vi "RT.vi"() -> ()   [LabVIEW 2017]
panel:
  in  "Inject error":bool
  out "Numeric":i32
  out "Boolean":bool
  in  "stop":bool
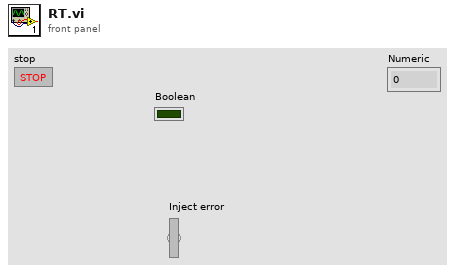
[diagram p1: front panel]
types:
  T1 = cluster{"source":string, "message":variant, "timestamp":timestamp}
  T2 = enum16{"open", "replace", "create", "open or create", "replace or create", "replace or create with confirmation"}
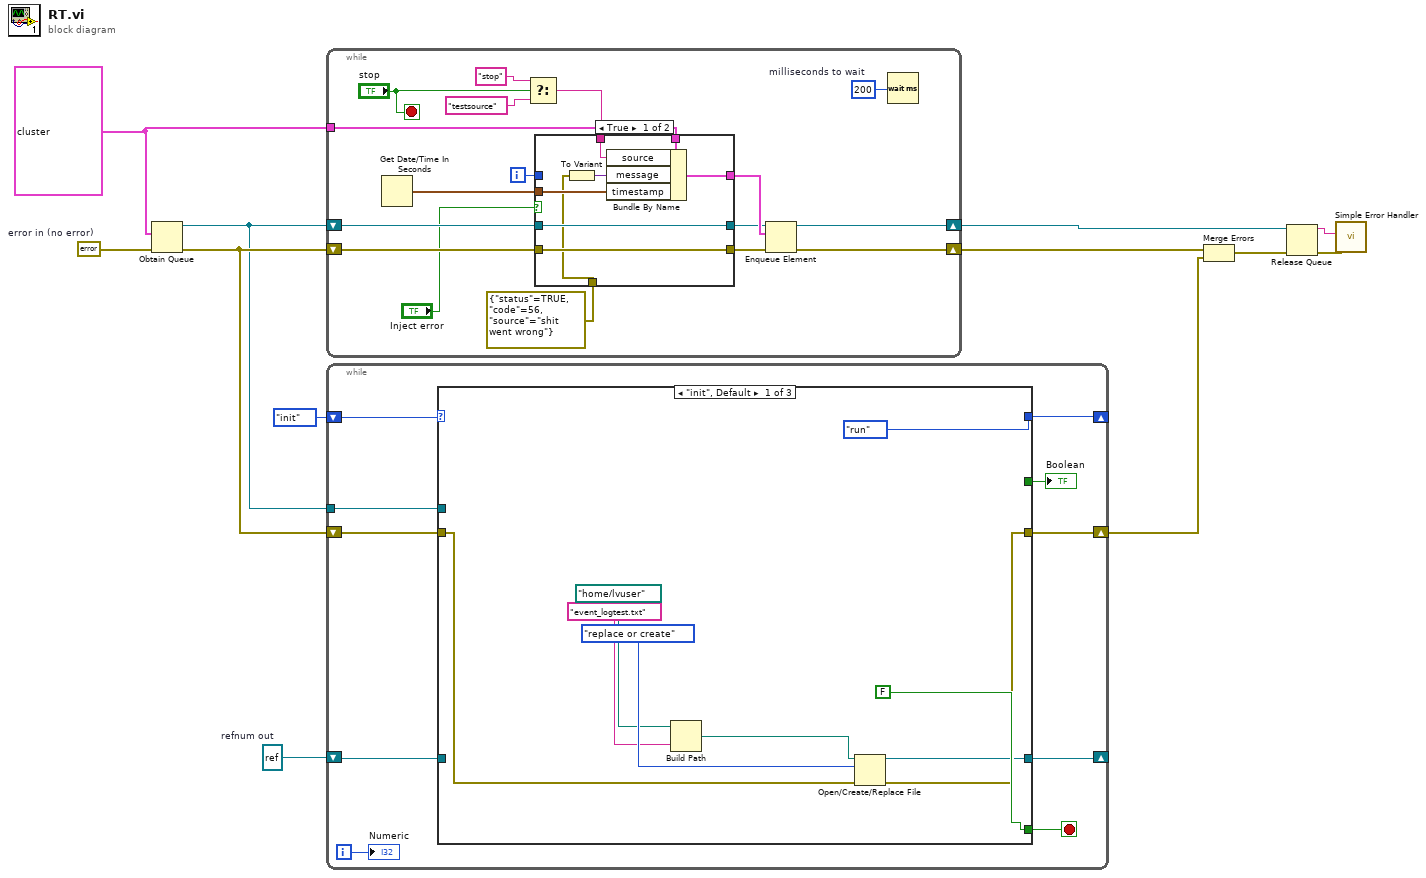
[diagram p0: block diagram]
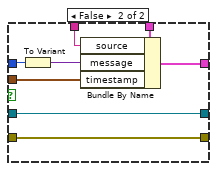
[diagram p2: hidden frame]
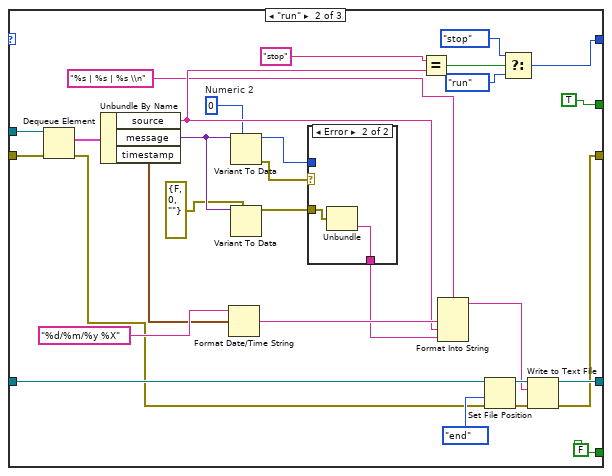
[diagram p3: hidden frame]
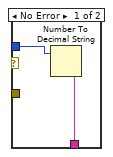
[diagram p4: hidden frame]
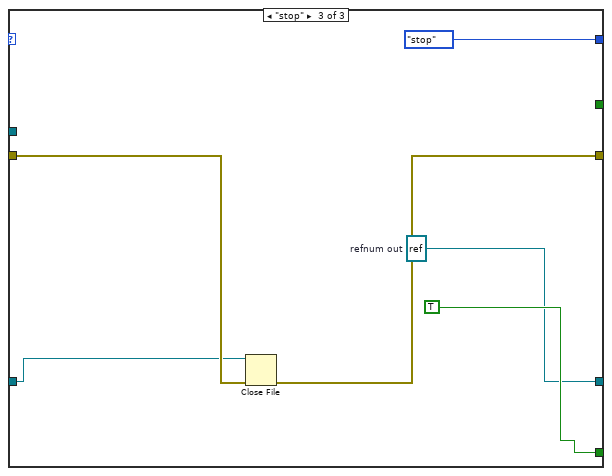
[diagram p5: hidden frame]
diagram:
  w7 = refnum<file> refnum  # refnum out
  w10 = T1 {"source"="", "message"=variant, "timestamp"=timestamp(0 s since 1904-01-01)}
  w12 = errorcluster {"status"=FALSE, "code"=0, "source"=""}  # error in (no error)
  n1 = Obtain Queue(element data type=w10, error in (no error)=w12) -> (queue out=w8:refnum<queue>, error out=w11:errorcluster)  [unwired: 3 in, 1 out]
  n2 = while {
    shift-right: [w27] -> w6
    shift-left: w11 -> [w17]
    shift-right: [w28] -> w3
    shift-left: w8 -> [w18]
    tunnel: w10 -> [w19]
    i -> [w20]
    stop <- "stop" stop-if-true
    w29 = u32 200  # milliseconds to wait
    n3 = Get Date/Time In Seconds() -> (seconds since 1Jan1904=w25:timestamp)
    n4 = Select(t="stop" ("source"), s="stop", f="testsource" ("source")) -> (s? t:f=w21:string)
    n5 = case shown="True" "Inject error" {
      tunnel: [w37 w45] -> w26
      tunnel: w25 -> [w36 w44]
      tunnel: w21 -> [w35 w43]
      tunnel: w20 -> [_ w42]
      tunnel: w19 -> [w33 w40]
      tunnel: w18 -> [w32 w39]
      tunnel: w17 -> [w31 w38]
      tunnel: [w32 w39] -> w16
      tunnel: [w31 w38] -> w15
      tunnel: errorcluster {"status"=TRUE, "code"=56, "source"="shit went wrong"} ("error constant") -> [w30 _]
      frame True {
        n6 = To Variant(anything=w30) -> (Variant=w34:variant)
        n7 = Bundle By Name(cluster=w33, "source"=w35, "message"=w34, "timestamp"=w36) -> (w37:T1)
      }
      frame False {
        n8 = To Variant(anything=w42) -> (Variant=w41:variant)
        n9 = Bundle By Name(cluster=w40, "source"=w43, "message"=w41, "timestamp"=w44) -> (w45:T1)
      }
    }
    n10 = Enqueue Element(queue=w16, element=w26, error in (no error)=w15) -> (queue out=w28:refnum<queue>, error out=w27:errorcluster)  [unwired: 1 in, 1 out]
    n11 = Wait (ms)(milliseconds to wait=w29) -> ()  [unwired: 1 out]
  }
  n12 = while {
    shift-right: [w50] -> w5
    shift-left: w11 -> [w52]
    shift-right: [w54] -> _
    shift-left: enum16{"init", "run", "stop"}."init" -> [w55]
    tunnel: w8 -> [w51]
    shift-right: [w49] -> _
    shift-left: w7 -> [w48]
    i -> [w46]
    stop <- w53 stop-if-true
    n13 = case shown="\"init\", Default" w55 {
      tunnel: [enum16{"init", "run", "stop"}."run" w87 enum16{"init", "run", "stop"}."stop"] -> w54
      tunnel: [FALSE FALSE TRUE] -> w53
      tunnel: w51 -> [_ w93 _]
      tunnel: w52 -> [w59 w92 w102]
      tunnel: [w58 w81 w100] -> w50
      tunnel: [w57 w82 w99] -> w49
      tunnel: w48 -> [_ w83 w101]
      tunnel: [_ TRUE _] -> w47
      frame "init", Default {
        n14 = Build Path(base path=path "/home/lvuser", name or relative path="event_logtest.txt") -> (appended path=w61:path)
        n15 = Open/Create/Replace File(file path (use dialog)=w61, error in=w59, operation (0:open)=T2."replace or create") -> (refnum out=w57:refnum<file>, error out=w58:errorcluster)  [unwired: 3 in, 1 out]
      }
      frame "run" {
        w70 = 0  # Numeric 2
        n16 = Dequeue Element(queue=w93, error in (no error)=w92) -> (element=w72:T1, error out=w74:errorcluster)  [unwired: 1 in, 2 out]
        n17 = Unbundle By Name(w72) -> ("source"=w77:string, "message"=w71:variant, "timestamp"=w79:timestamp)
        n18 = Format Date/Time String(time format string (%c)="%d/%m/%y %X", seconds (now)=w79) -> (date/time string=w78:string)  [unwired: 1 in]
        n19 = Variant To Data(type=w70, Variant=w71) -> (data=w69:i32, error out=w65:errorcluster)  [unwired: 1 in]
        n20 = Variant To Data(type=errorcluster {"status"=FALSE, "code"=0, "source"=""} ("error constant"), Variant=w71) -> (data=w66:errorcluster)  [unwired: 1 in, 1 out]
        n21 = case shown="Error" w65 {
          tunnel: w69 -> [w96 _]
          tunnel: [w95 w97] -> w68
          tunnel: w66 -> [_ w98]
          frame No Error {
            n22 = Number To Decimal String(number=w96) -> (decimal integer string=w95:string)  [unwired: 1 in]
          }
          frame Error {
            n23 = Unbundle(w98) -> ("source"=w97:string)  [unwired: 2 out]
          }
        }
        n24 = Equal?(x="stop" ("source"), y=w77) -> (x = y?=w90:bool)
        n25 = Format Into String(format string="%s | %s | %s \\n", w78, w77, w68) -> (resulting string=w76:string)  [unwired: 2 in, 1 out]
        n26 = Set File Position(refnum=w83, from (0:start)=enum16{"start", "end", "current"}."end", error in=w74) -> (refnum out=w84:refnum<file>, error out=w86:errorcluster)  [unwired: 1 in]
        n27 = Select(t=enum16{"init", "run", "stop"}."stop", s=w90, f=enum16{"init", "run", "stop"}."run") -> (s? t:f=w87:enum16{"init", "run", "stop"})
        n28 = Write to Text File(file (use dialog)=w84, text=w76, error in=w86) -> (refnum out=w82:refnum<file>, error out=w81:errorcluster)  [unwired: 1 in, 1 out]
      }
      frame "stop" {
        w99 = refnum<file> refnum  # refnum out
        n29 = Close File(refnum=w101, error in=w102) -> (error out=w100:errorcluster)  [unwired: 1 out]
      }
    }
    "Boolean" <- w47
    "Numeric" <- w46
  }
  n30 = Merge Errors(w6, w5) -> (w4:errorcluster)
  n31 = Release Queue(queue=w3, error in (no error)=w4) -> (queue name=w2:string, error out=w1:errorcluster)  [unwired: 1 in, 1 out]
  n32 = call <vilib>:"Simple Error Handler.vi"("error source (\" \")"=w2, "error in (no error)"=w1) -> ()  [unwired: 3 in, 5 out]
